vi "retrieve.vi"(8 "error in (no error)":errorcluster, 11 "DL090215DataCollection in":refnum<class "DataCollectionMG091001IntrinsicImaging.lvclass">) -> (0 "error out":errorcluster, 3 "DL090215DataCollection out":refnum<class "DataCollectionMG091001IntrinsicImaging.lvclass">)   [LabVIEW 2010, in "DataCollectionMG091001IntrinsicImaging.lvclass"]
uses:
  DataCollectionMG091001IntrinsicImaging.lvclass
  DataCollectionMG091001IntrinsicImaging.lvclass/DataCollectionMG091001IntrinsicImaging.ctl
  common/classes/Image/Image/storage_mode.ctl
  common/classes/ImageCollection/ImageCollection/ImageCollection.lvclass
  common/classes/ImageCollection/ImageCollection/add_mode_enum.ctl
  common/classes/Image/Image/Image.lvclass
  common/classes/ErrorController/ErrorController/class_data.vi
  common/classes/ErrorController/ErrorController/ErrorController.lvclass
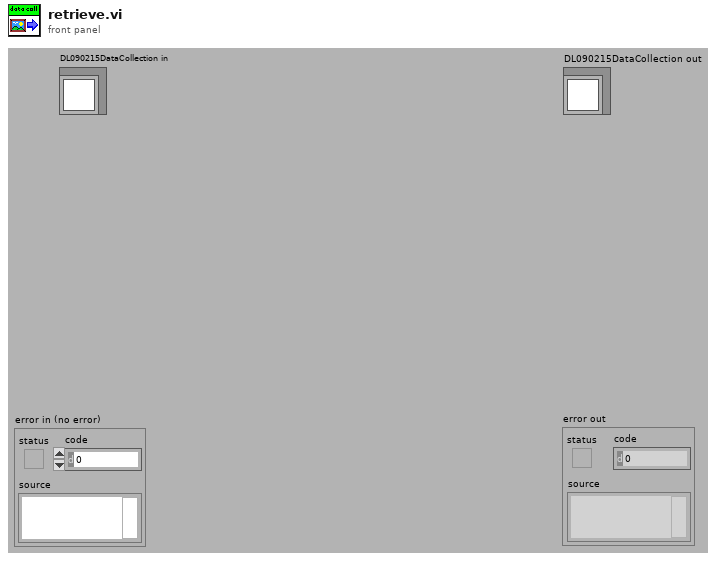
[diagram p1: front panel]
types:
  T1 = typedef "Image.lvclass/storage_mode.ctl" = enum16{"RAM", "disk"}
  T2 = typedef "ImageCollection.lvclass/add_mode_enum.ctl" = enum16{"instance", "copy"}
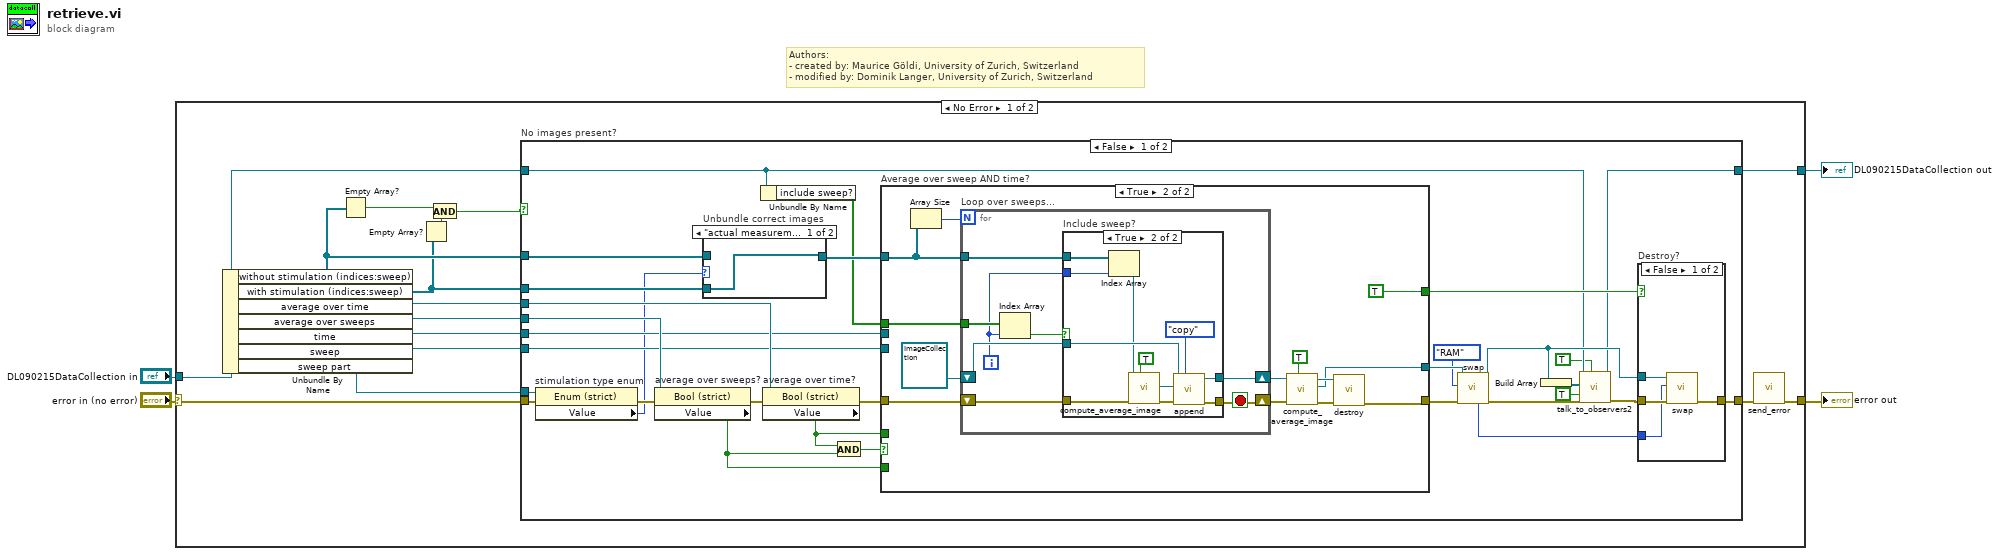
[diagram p0: block diagram]
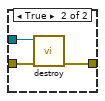
[diagram p2: hidden frame]
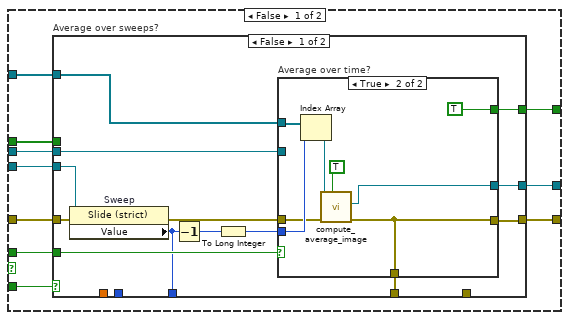
[diagram p3: hidden frame]
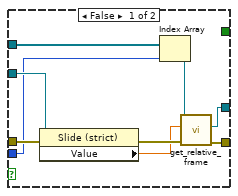
[diagram p4: hidden frame]
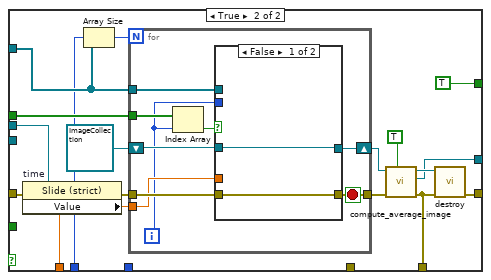
[diagram p5: hidden frame]
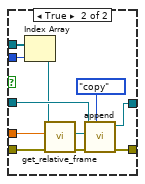
[diagram p6: hidden frame]
diagram:
  # "Authors: \n- created by: Maurice Göldi, University of Zurich, Switzerland\n- modified by: Dominik Langer, University of Zurich, Switzerland"
  n1 = case shown="No Error" "error in (no error)" {
    selector: "error in (no error)" -> [w15 w175]
    tunnel: [w9 w175] -> w3
    tunnel: [w6 w174] -> w2
    tunnel: "DL090215DataCollection in" -> [w14 w174]
    frame No Error {
      n2 = Unbundle By Name(w14) -> ("without stimulation (indices:sweep)"=w12:refnum<class "ImageCollection.lvclass">[], "with stimulation (indices:sweep)"=w11:refnum<class "ImageCollection.lvclass">[], "average over time"=w18:refnum<vi>, "average over sweeps"=w19:refnum<vi>, "time"=w17:refnum<vi>, "sweep"=w16:refnum<vi>, "sweep part"=w13:refnum<vi>)
      n3 = Empty Array?(array=w12) -> (empty?=w7:bool)
      n4 = Empty Array?(array=w11) -> (empty?=w8:bool)
      n5 = And(x=w7, y=w8) -> (x .and. y?=w10:bool)
      n6 = case "No images present?" shown="False" w10 {
        tunnel: w19 -> [w50 _]
        tunnel: w18 -> [w47 _]
        tunnel: w17 -> [w46 _]
        tunnel: w16 -> [w45 _]
        tunnel: w15 -> [w42 w172]
        tunnel: [w31 w172] -> w5
        tunnel: w14 -> [w24 w173]
        tunnel: w13 -> [w36 _]
        tunnel: w12 -> [w35 _]
        tunnel: w11 -> [w34 _]
        tunnel: [w23 w173] -> w6
        frame False {
          n7 = property on="stimulation type enum" class="Enum (strict)"(reference=w36, error in=w42) -> (error out=w41:errorcluster, "Value"=w28:enum16{"actual measurement", "control"})  [unwired: 1 out]
          n8 = property on="average over sweeps?" class="Bool (strict)"(reference=w50, error in=w41) -> (error out=w48:errorcluster, "Value"=w30:bool)  [unwired: 1 out]
          n9 = case "Unbundle correct images" shown="\"actual measurement\", Default" w28 {
            tunnel: [w170 w171] -> w49
            tunnel: w34 -> [w170 _]
            tunnel: w35 -> [_ w171]
            frame "actual measurement", Default {
            }
            frame "control" {
            }
          }
          n10 = Unbundle By Name(w24) -> ("include sweep?"=w27:bool[])
          n11 = property on="average over time?" class="Bool (strict)"(reference=w47, error in=w48) -> (error out=w33:errorcluster, "Value"=w29:bool)  [unwired: 1 out]
          n12 = And(x=w29, y=w30) -> (x .and. y?=w43:bool)
          n13 = case "Average over sweep AND time?" shown="True" w43 {
            tunnel: w49 -> [w67 w142]
            tunnel: w30 -> [w66 _]
            tunnel: w33 -> [w65 w147]
            tunnel: w29 -> [w64 _]
            tunnel: w46 -> [w63 _]
            tunnel: w45 -> [w62 _]
            tunnel: [w61 w143] -> w44
            tunnel: [w60 w139] -> w32
            tunnel: w27 -> [w59 w141]
            tunnel: [w58 TRUE] -> w40
            frame False {
              n14 = case "Average over sweeps?" shown="False" w66 {
                tunnel: w67 -> [w76 w103]
                tunnel: w65 -> [w80 w113]
                tunnel: [w74 w108] -> w60
                tunnel: [w73 w106] -> w61
                tunnel: w64 -> [w78 _]
                tunnel: w63 -> [w75 w112]
                tunnel: w62 -> [w77 _]
                tunnel: w59 -> [_ w102]
                tunnel: [w70 TRUE] -> w58
                tunnel: [_ w100] -> _
                tunnel: [w69 _] -> _
                tunnel: [_ w99] -> _
                tunnel: [_ w98] -> _
                tunnel: [w68 _] -> _
                frame False {
                  n15 = property on="Sweep" class="Slide (strict)"(reference=w77, error in=w80) -> (error out=w79:errorcluster, "Value"=w68:i32)  [unwired: 1 out]
                  n16 = Decrement(x=w68) -> (x-1=w72:i32)
                  n17 = To Long Integer(number=w72) -> (32bit integer=w71:i32)
                  n18 = case "Average over time?" shown="True" w78 {
                    tunnel: w79 -> [w89 w95]
                    tunnel: w71 -> [w81 w96]
                    tunnel: w76 -> [w87 w97]
                    tunnel: w75 -> [w88 _]
                    tunnel: [w83 w90] -> w74
                    tunnel: [w82 w92] -> w73
                    tunnel: [_ TRUE] -> w70
                    tunnel: [_ w90] -> w69
                    frame False {
                      n19 = property class="Slide (strict)"(reference=w88, error in=w89) -> (error out=w86:errorcluster, "Value"=w84:dbl[unit])  [unwired: 1 out]
                      n20 = Index Array(array=w87, index=w81) -> (element=w85:refnum<class "ImageCollection.lvclass">)
                      n21 = call-dynamic "get_relative_frame.vi"("error in (no error)"=w86, "relative time"=w84, "ImageCollection in"=w85) -> ("error out"=w83:errorcluster, "frame"=w82:refnum<class "Image.lvclass">)  [unwired: 5 in, 2 out]
                    }
                    frame True {
                      n22 = Index Array(array=w97, index=w96) -> (element=w94:refnum<class "ImageCollection.lvclass">)
                      n23 = call-dynamic "compute_average_image.vi"("all?"=TRUE, "error in (no error)"=w95, "ImageCollection in"=w94) -> ("error out"=w90:errorcluster, "averaged image"=w92:refnum<class "Image.lvclass">)  [unwired: 6 in, 1 out]
                    }
                  }
                }
                frame True {
                  n24 = property on="time" class="Slide (strict)"(reference=w112, error in=w113) -> (error out=w104:errorcluster, "Value"=w99:dbl[unit])  [unwired: 1 out]
                  n25 = Array Size(array=w103) -> (size(s)=w98:i32)
                  n26 = for {
                    N: w98 -> [_]
                    tunnel: w103 -> [w118]
                    tunnel: w99 -> [w121]
                    shift-right: [w119] -> w110
                    shift-left: refnum<class "ImageCollection.lvclass"> refnum ("ImageCollection.lvclass") -> [w120]
                    tunnel: w102 -> [w116]
                    tunnel: w104 -> [w122]
                    tunnel: [w114] -> w111
                    i -> [w115]
                    stop <- w114 stop-if-true
                    n27 = Index Array(array=w116, index=w115) -> (element=w117:bool)
                    n28 = case shown="False" w117 {
                      tunnel: w122 -> [w124 w135]
                      tunnel: w121 -> [_ w134]
                      tunnel: w120 -> [w123 w132]
                      tunnel: [w123 w130] -> w119
                      tunnel: [w124 w129] -> w114
                      tunnel: w118 -> [_ w127]
                      tunnel: w115 -> [_ w126]
                      frame False {
                      }
                      frame True {
                        n29 = Index Array(array=w127, index=w126) -> (element=w125:refnum<class "ImageCollection.lvclass">)
                        n30 = call-dynamic "get_relative_frame.vi"("error in (no error)"=w135, "relative time"=w134, "ImageCollection in"=w125) -> ("error out"=w133:errorcluster, "frame"=w131:refnum<class "Image.lvclass">)  [unwired: 5 in, 2 out]
                        n31 = call-dynamic "append.vi"("add mode"=add_mode_enum."copy", "error in (no error)"=w133, "Image.lvclass"=w131, "ImageCollection in"=w132) -> ("error out"=w129:errorcluster, "ImageCollection out"=w130:refnum<class "ImageCollection.lvclass">)  [unwired: 5 in, 1 out]
                      }
                    }
                  }
                  n32 = call-dynamic "compute_average_image.vi"("all?"=TRUE, "error in (no error)"=w111, "ImageCollection in"=w110) -> ("error out"=w100:errorcluster, "averaged image"=w106:refnum<class "Image.lvclass">, "ImageCollection out"=w107:refnum<class "ImageCollection.lvclass">)  [unwired: 6 in]
                  n33 = call-dynamic "destroy.vi"("error in (no error)"=w100, "ImageCollection in"=w107) -> ("error out"=w108:errorcluster)  [unwired: 8 in, 1 out]
                }
              }
            }
            frame True {
              n34 = Array Size(array=w142) -> (size(s)=w138:i32)
              n35 = for "Loop over sweeps..." {
                N: w138 -> [_]
                tunnel: w142 -> [w153]
                shift-right: [w149] -> w136
                shift-left: w147 -> [w156]
                shift-right: [w154] -> w146
                shift-left: refnum<class "ImageCollection.lvclass"> refnum ("ImageCollection.lvclass") -> [w155]
                tunnel: w141 -> [w152]
                i -> [w151]
                stop <- w149 stop-if-true
                n36 = Index Array(array=w152, index=w151) -> (element=w150:bool)
                n37 = case "Include sweep?" shown="True" w150 {
                  tunnel: w156 -> [w158 w169]
                  tunnel: w155 -> [w157 w166]
                  tunnel: [w158 w163] -> w149
                  tunnel: [w157 w162] -> w154
                  tunnel: w153 -> [_ w161]
                  tunnel: w151 -> [_ w159]
                  frame False {
                  }
                  frame True {
                    n38 = Index Array(array=w161, index=w159) -> (element=w160:refnum<class "ImageCollection.lvclass">)
                    n39 = call-dynamic "compute_average_image.vi"("all?"=TRUE, "error in (no error)"=w169, "ImageCollection in"=w160) -> ("error out"=w167:errorcluster, "averaged image"=w165:refnum<class "Image.lvclass">)  [unwired: 6 in, 1 out]
                    n40 = call-dynamic "append.vi"("add mode"=add_mode_enum."copy", "error in (no error)"=w167, "Image.lvclass"=w165, "ImageCollection in"=w166) -> ("error out"=w163:errorcluster, "ImageCollection out"=w162:refnum<class "ImageCollection.lvclass">)  [unwired: 5 in, 1 out]
                  }
                }
              }
              n41 = call-dynamic "compute_average_image.vi"("all?"=TRUE, "error in (no error)"=w136, "ImageCollection in"=w146) -> ("error out"=w137:errorcluster, "averaged image"=w143:refnum<class "Image.lvclass">, "ImageCollection out"=w144:refnum<class "ImageCollection.lvclass">)  [unwired: 6 in]
              n42 = call-dynamic "destroy.vi"("error in (no error)"=w137, "ImageCollection in"=w144) -> ("error out"=w139:errorcluster)  [unwired: 8 in, 1 out]
            }
          }
          n43 = call-dynamic "swap.vi"("error in (no error)"=w32, "storage type target"=storage_mode."RAM", "Image in"=w44) -> ("error out"=w26:errorcluster, "Image out"=w37:refnum<class "Image.lvclass">, "previous storage mode"=w38:T1)  [unwired: 6 in]
          n44 = Build Array(w37) -> (w25:refnum<class "Image.lvclass">[])
          n45 = call-dynamic "talk_to_observers2.vi"("force sending?"=TRUE, "error in (no error)"=w26, "image finished?"=TRUE, "image (channels)"=w25, "GenericToplevelComponent in"=w24) -> ("error out"=w22:errorcluster, "GenericToplevelComponent out"=w23:refnum<class "DataCollectionMG091001IntrinsicImaging.lvclass">)  [unwired: 5 in]
          n46 = case "Destroy?" shown="False" w40 {
            tunnel: [w54 w55] -> w31
            tunnel: w22 -> [w53 w57]
            tunnel: w38 -> [w52 _]
            tunnel: w37 -> [w51 w56]
            frame False {
              n47 = call-dynamic "swap.vi"("error in (no error)"=w53, "storage type target"=w52, "Image in"=w51) -> ("error out"=w54:errorcluster)  [unwired: 6 in, 2 out]
            }
            frame True {
              n48 = call-dynamic "destroy.vi"("error in (no error)"=w57, "Image in"=w56) -> ("error out"=w55:errorcluster)  [unwired: 8 in, 1 out]
            }
          }
        }
        frame True {
          # "Don't do anything in this case..."
        }
      }
      n49 = call "send_error.vi"("error in (no error)"=w5) -> ("error out"=w9:errorcluster)  [unwired: 10 in]
    }
    frame Error {
    }
  }
  "error out" <- w3
  "DL090215DataCollection out" <- w2
